vi "PXI-Channel Name to Physical Channel.vi"(0 "Channel Name":string, 11 "error in (no error)":errorcluster) -> (4 "Physical Channel":tag, 15 "error out":errorcluster)   [LabVIEW 2020]
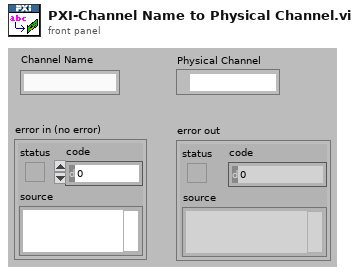
[diagram p1: front panel]
types:
  T1 = cluster{"DAQChan to PhysDev":i32[][], "PhysDev to DAQChan":i32[][]}
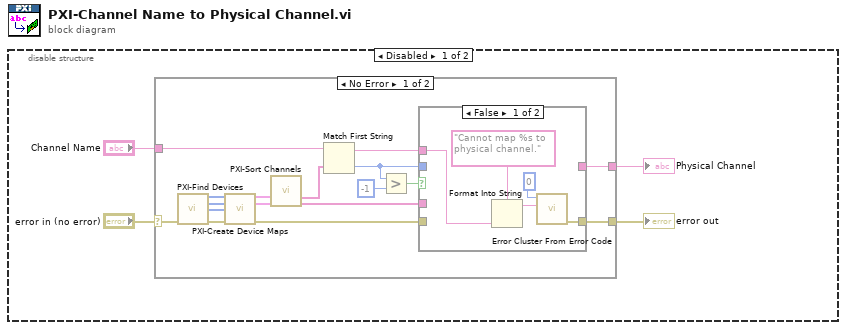
[diagram p0: block diagram]
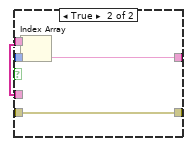
[diagram p2: hidden frame]
diagram:
  n1 = disable-structure shown="Disabled" {
    frame Disabled {
      n2 = case shown="No Error" "error in (no error)" {
        selector: "error in (no error)" -> [w6 w31]
        tunnel: "Channel Name" -> [w14 _]
        tunnel: [w8 w31] -> w3
        tunnel: [w7 _] -> w2
        frame No Error {
          n3 = call "PXI-Find Devices.vi"("error in (no error)"=w6) -> ("Num AO"=w19:i32[], "Num AI"=w18:i32[], "Slot Num"=w21:u32[], "error out"=w20:errorcluster)  [unwired: 11 in]
          n4 = call "PXI-Create Device Maps.vi"("Num AO"=w19, "Num AI"=w18, "Slot Num"=w21, "error in (no error)"=w20) -> ("AO Map"=w17:T1, "AI Map"=w16:T1, "error out"=w9:errorcluster)  [unwired: 9 in]
          n5 = call "PXI-Sort Channels.vi"("AO Map"=w17, "AI Map"=w16) -> ("Sorted channel names"=w15:string[], "Sorted physical channels"=w10:tag[])  [unwired: 12 in]
          n6 = Match First String(2:w15, 3:w14) -> (0:w11:i32, 1:w5:string)
          n7 = Greater?(x=w11, y=-1) -> (0:w12:bool)
          n8 = case shown="False" w12 {
            tunnel: w11 -> [_ w30]
            tunnel: w10 -> [_ w29]
            tunnel: [_ w28] -> w7
            tunnel: w9 -> [_ w27]
            tunnel: [w26 w27] -> w8
            tunnel: w5 -> [w22 _]
            frame False {
              n9 = Format Into String(format string="Cannot map %s to physical channel.", w22) -> (resulting string=w25:string)  [unwired: 2 in, 1 out]
              n10 = call <vilib>:"Error Cluster From Error Code.vi"("error message (\"\")"=w25, "error code (0)"=0) -> ("error out"=w26:errorcluster)  [unwired: 7 in]
            }
            frame True {
              n11 = Index Array(array=w29, index=w30) -> (element=w28:tag)
            }
          }
        }
        frame Error {
        }
      }
      "error out" <- w3
      "Physical Channel" <- w2
    }
    frame Enabled {
    }
  }
